vi "Test RD Retrieval.vi"() -> ()   [LabVIEW 2015]
uses:
  <vilib>/eio/EIOGrowableMethodNode/genericMethod/EIOGrowableMethodNode.xnode
  <vilib>/rvi/eio/nirviErrorMerge/nirviErrorMerge.xnode
  <vilib>/rvi/eio/nirviEIOMethodImplementation/nirviEIOMethodImplementation.xnode
  <vilib>/rvi/eio/common/nirviEmuTemplateMethod_errors.vi
  <vilib>/rvi/eio/common/nirviEmuClasses.ctl
  <vilib>/rvi/DataTransferAndStorage/Container/XNode/niFpgaContainer.xnode
  <vilib>/rvi/eio/common/nirviEmuTemplateMethod_noerrors.vi
  <vilib>/rvi/interface/RandomDataEmulation/nirviRandomDataFpgaReadWriteTemplate.vi
  <vilib>/eio/EIONode/EIONode.xnode
  <vilib>/rvi/Memory/Memory_Emulation/nirvimemoryFastEmulation.vi
  <vilib>/rvi/Memory/Memory_Emulation/nirvimemoryEmulation.vi
  <vilib>/rvi/FIFO/Fifo_Resource/nirvififoEmulationClear.vi
  <vilib>/rvi/FIFO/Fifo_Resource/nirvififoEmulationGetNumberOfElementsToRead.vi
  <vilib>/rvi/FIFO/Fifo_Resource/nirvififoEmulationRead.vi
  <vilib>/rvi/FIFO/Fifo_Resource/nirvififoEmulationWrite.vi
  <vilib>/rvi/FIFO/Fifo_Resource/niFpgaFifoEmulationRefIn.vi
panel:
  in  "Num2Acq":u16
  in  "DC":u16=500
  in  "TotNumSamp":u16=1000
  in  "Stop":bool
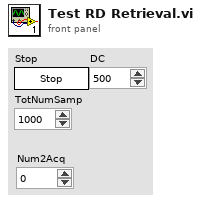
[diagram p1: front panel]
types:
  T1 = typedef "nirviEmuClasses.ctl" = enum16{"IO Read", "IO Write", "Method", "Property Read", "Property Write"}
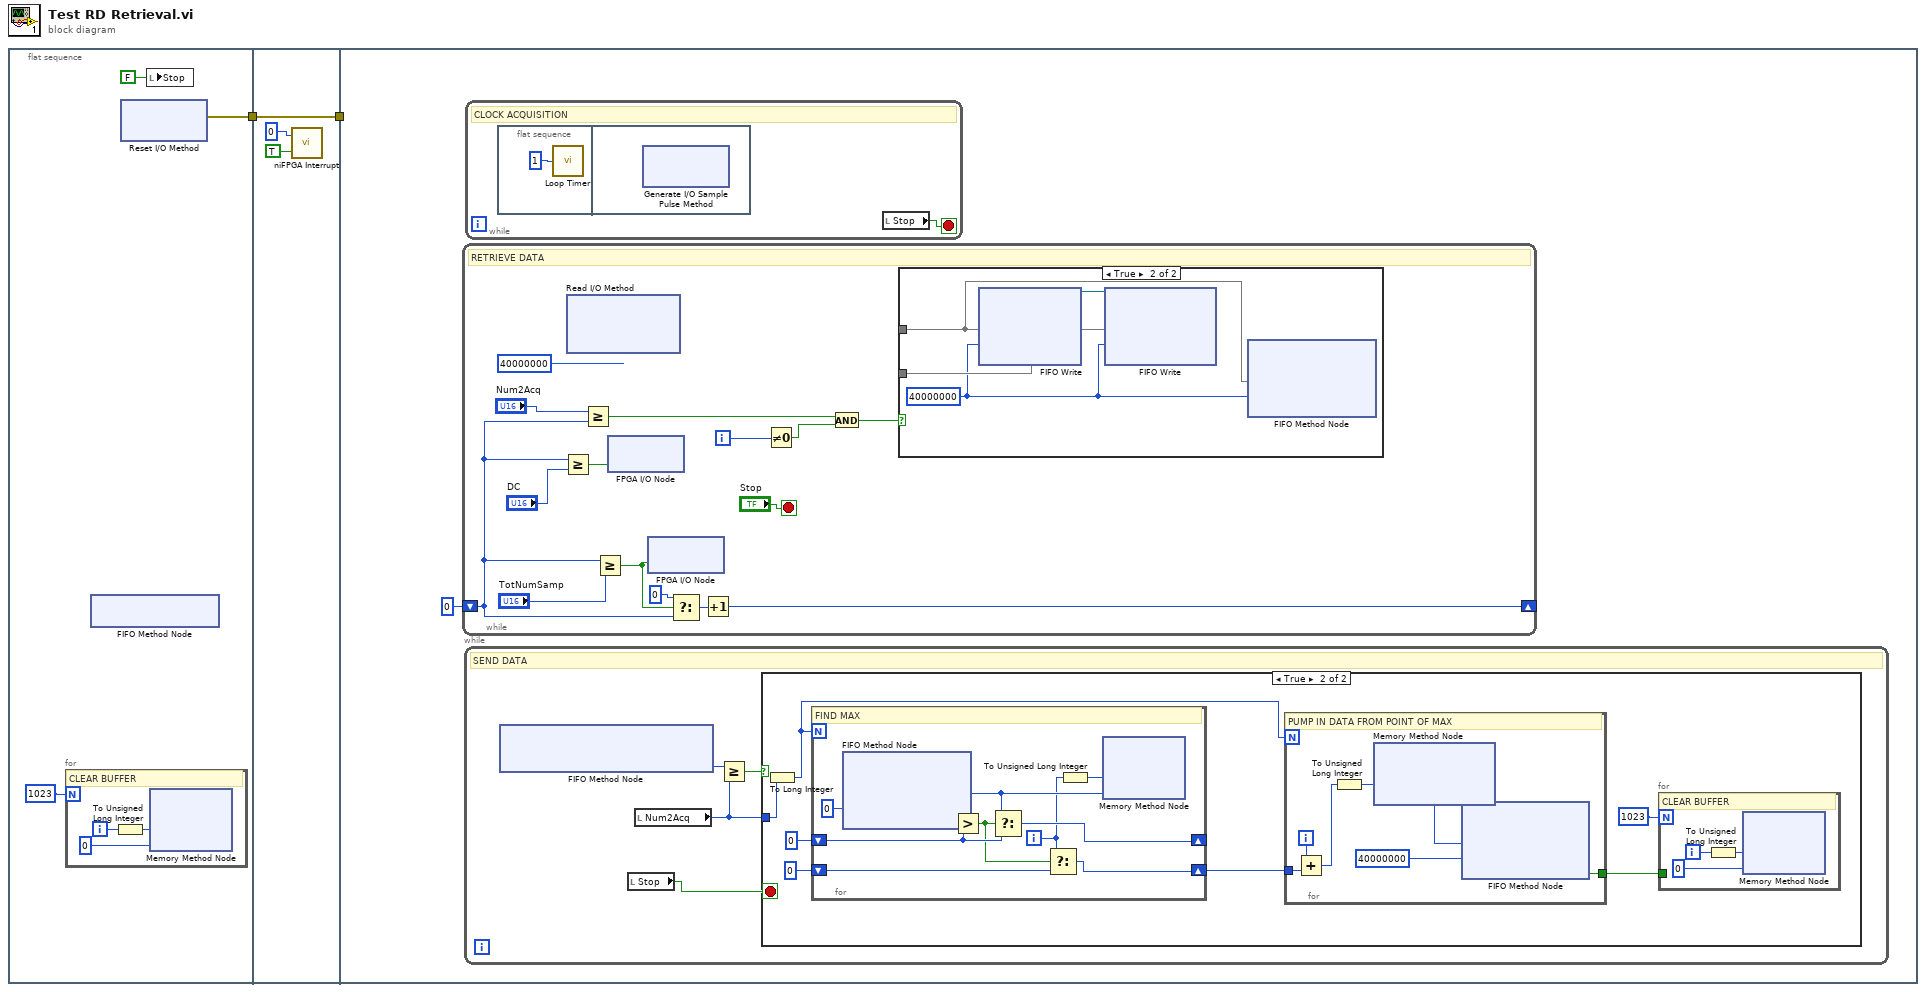
[diagram p0: block diagram]
diagram:
  n1 = flat-sequence {
    tunnel: [w5] -> w2
    tunnel: w2 -> [w55]
    tunnel: [w55] -> w1
    tunnel: w1 -> [_]
    frame #0 {
      n2 = for {
        N: 1023 -> [_]
        i -> [w7]
        # "CLEAR BUFFER"
        n3 = To Unsigned Long Integer(number=w7) -> (unsigned 32bit integer=w6:u32)
        n4 = xnode ("Memory Method Node")("Address"=w6, "Data"=i16 0) -> ()  [unwired: 1 in, 1 out]
      }
      n5 = xnode ("FIFO Method Node")() -> ()  [unwired: 1 in, 1 out]
      n6 = xnode "Reset I/O Method"() -> ("error out"=w5:errorcluster)  [unwired: 1 in]
      n7 = local write "Stop"(FALSE ("Stop")) -> ()
    }
    frame #1 {
      n8 = call <vilib>:"niFPGA Interrupt.vi"("Wait Until Cleared (F)"=TRUE ("Wait Until Cleared"), "IRQ Number (0)"=u8 0 ("IRQ Number")) -> ()  [unwired: 1 in]
    }
    frame #2 {
      n9 = while {
        shift-right: [w100] -> _
        shift-left: u16 0 -> [w102]
        i -> [w98]
        stop <- "Stop" stop-if-true
        # "RETRIEVE DATA"
        n10 = Greater Or Equal?(x=w102, y="DC") -> (x >= y?=w103:bool)
        n11 = xnode "Read I/O Method"(40000000 ("Timeout")) -> ()  [unwired: 1 in, 1 out]
        n12 = Greater Or Equal?(x="Num2Acq", y=w102) -> (x >= y?=w97:bool)
        n13 = Greater Or Equal?(x=w102, y="TotNumSamp") -> (x >= y?=w106:bool)
        n14 = xnode "FPGA I/O Node"("Diode"=w103) -> ()  [unwired: 1 in, 1 out]
        n15 = xnode "FPGA I/O Node"("CRDS"=w106) -> ()  [unwired: 1 in, 1 out]
        n16 = Select(t=u16 0 ("Number of Samples"), s=w106, f=w102) -> (s? t:f=w101:u16)
        n17 = Increment(x=w101) -> (x+1=w100:u16)
        n18 = Not Equal To 0?(x=w98) -> (x != 0?=w96:bool)
        n19 = And(x=w97, y=w96) -> (x .and. y?=w95:bool)
        n20 = case shown="True" w95 {
          tunnel: [_ w113] -> w105
          tunnel: [_ w114] -> w104
          frame False {
          }
          frame True {
            w112 = 40000000 ("Timeout")
            n21 = xnode ("FIFO Write")("Element"=w113, "Timeout"=w112) -> ("FIFO Out"=w115:refnum<k21>)  [unwired: 2 in, 2 out]
            n22 = xnode ("FIFO Write")("Element"=w114, "Timeout"=w112, "FIFO In"=w115) -> ()  [unwired: 1 in, 3 out]
            n23 = xnode ("FIFO Method Node")("Element"=w113, "Timeout"=w112) -> ()  [unwired: 1 in, 2 out]
          }
        }
      }
      n24 = while {
        stop <- w57 stop-if-true
        # "SEND DATA"
        n25 = xnode ("FIFO Method Node")() -> ("Number of Elements to Read"=w60:u32)  [unwired: 1 in, 1 out]
        n26 = local read "Stop"() -> (w57:bool)
        n27 = local read "Num2Acq"() -> (w58:u16)
        n28 = Greater Or Equal?(x=w60, y=w58) -> (x >= y?=w59:bool)
        n29 = case shown="True" w59 {
          tunnel: w58 -> [_ w62]
          frame False {
          }
          frame True {
            n30 = To Long Integer(number=w62) -> (32bit integer=w61:i32)
            n31 = for {
              N: w61 -> [_]
              shift-right: [w83] -> _
              shift-left: i16 0 ("Element") -> [w84]
              shift-right: [w80] -> w65
              shift-left: 0 -> [w81]
              i -> [w79]
              # "FIND MAX"
              n32 = xnode ("FIFO Method Node")("Timeout"=0) -> ("Element"=w85:i16)  [unwired: 1 in, 2 out]
              n33 = Greater?(x=w85, y=w84) -> (0:w82:bool)
              n34 = Select(t=w85, s=w82, f=w84) -> (s? t:f=w83:i16)
              n35 = Select(t=w79, s=w82, f=w81) -> (s? t:f=w80:i32)
              n36 = To Unsigned Long Integer(number=w79) -> (unsigned 32bit integer=w78:u32)
              n37 = xnode ("Memory Method Node")("Address"=w78, "Data"=w85) -> ()  [unwired: 1 in, 1 out]
            }
            n38 = for {
              N: w61 -> [_]
              tunnel: w65 -> [w76]
              tunnel: [w73] -> w63
              i -> [w77]
              # "PUMP IN DATA FROM POINT OF MAX"
              n39 = Add(x=w77, y=w76) -> (x+y=w72:i32)
              n40 = To Unsigned Long Integer(number=w72) -> (unsigned 32bit integer=w71:u32)
              n41 = xnode ("Memory Method Node")("Address"=w71) -> ("Data"=w74:i16)  [unwired: 1 in, 1 out]
              n42 = xnode ("FIFO Method Node")("Element"=w74, "Timeout"=40000000) -> ("Timed Out?"=w73:bool)  [unwired: 1 in, 1 out]
            }
            n43 = for {
              N: 1023 -> [_]
              tunnel: w63 -> [_]
              i -> [w69]
              # "CLEAR BUFFER"
              n44 = To Unsigned Long Integer(number=w69) -> (unsigned 32bit integer=w68:u32)
              n45 = xnode ("Memory Method Node")("Address"=w68, "Data"=i16 0) -> ()  [unwired: 1 in, 1 out]
            }
          }
        }
      }
      n46 = while {
        stop <- w87 stop-if-true
        # "CLOCK ACQUISITION"
        n47 = flat-sequence {
          frame #0 {
            n48 = call "Loop Timer"("Count(uSec)"=u32 1 ("Count(Ticks)")) -> ()  [unwired: 1 out]
          }
          frame #1 {
            n49 = xnode "Generate I/O Sample Pulse Method"() -> ()  [unwired: 1 in, 1 out]
          }
        }
        n50 = local read "Stop"() -> (w87:bool)
      }
    }
  }
